vi "test-quintic-spline-05.vi"() -> (3 "Test Passed":bool)   [LabVIEW 2019]
uses:
  <vilib>/Rock Robotics/WPI/ThirdParty/JAS_Junk/TrajLib/POSEwCURVATURE.ctl
  <vilib>/Rock Robotics/WPI/ThirdParty/JAS_Junk/TrajLib/POSE2D.ctl
  <vilib>/Rock Robotics/WPI/ThirdParty/JAS_Junk/TrajLib/TRANSLATION2D.ctl
  <vilib>/Rock Robotics/WPI/ThirdParty/JAS_Junk/TrajLib/ROTATION2D.ctl
  <vilib>/Rock Robotics/WPI/ThirdParty/JAS_Junk/TrajLib/Rotation_CreateAngle.vi
  <vilib>/Rock Robotics/WPI/ThirdParty/JAS_Junk/TrajLib/Translation_Create.vi
  <vilib>/Rock Robotics/WPI/ThirdParty/JAS_Junk/TrajLib/Util_CalcDist.vi
  <vilib>/Rock Robotics/WPI/ThirdParty/JAS_Junk/TrajLib/Trajectory_Library.lvlib
panel:
  out "XY Graph":cluster{dbl[], dbl[]}(graph)
  out "Numb\nWaypoints":i32
  out "All Interior \nwayPoints\nFound (True)":bool
  out "end rot = 0":dbl
  out "end y = 0":dbl
  out "end x = 0":dbl
  out "start rot = 0":dbl
  out "start y = 0":dbl
  out "start x = 0":dbl
  out "max dtheta < 0.0872":dbl
  out "max dy < 0.00127":dbl
  out "max dx  < 0.127":dbl
  out "Overall Error":errorcluster
  out "Elements":i32
  out "Create Spline Error":errorcluster
  out "SplinePoses\nWCurve":T1[](array[typedef]) {"POSE"."ROTATION"."SIN" format="%13.4f"; "POSE"."ROTATION"."COS" format="%13.4f"; "POSE"."ROTATION"."VALUE" format="%13.4f"; "POSE"."TRANSLATION"."Y" format="%14.3f"; "POSE"."TRANSLATION"."X" format="%14.3f"}
  out "Elapsed Time":dbl
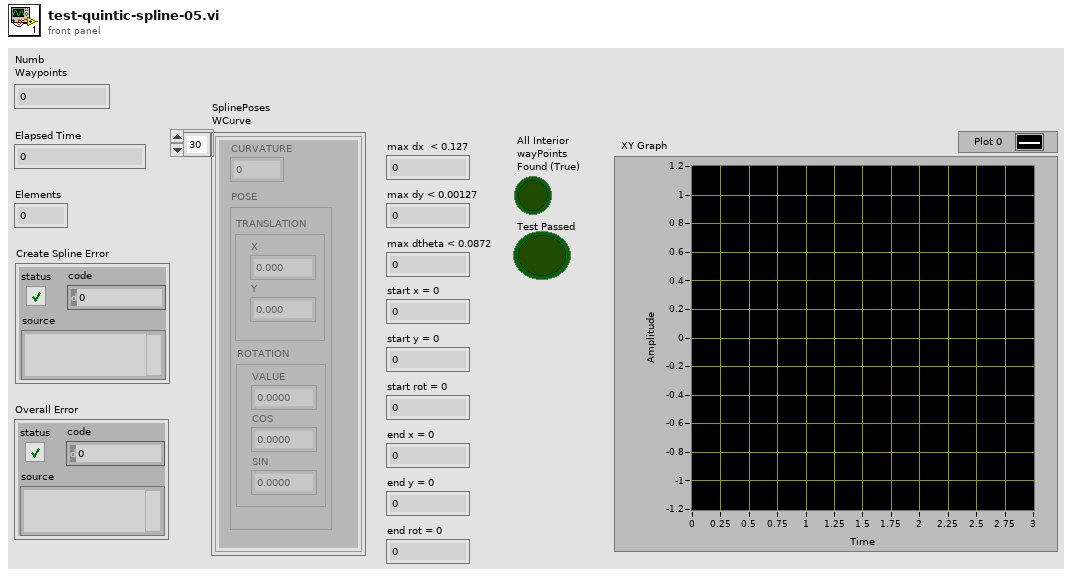
[diagram p1: front panel]
types:
  T1 = typedef "Trajectory_Library.lvlib/POSEwCURVATURE.ctl" = cluster{"CURVATURE":dbl, "POSE":T2}
  T2 = typedef "Trajectory_Library.lvlib/POSE2D.ctl" = cluster{"TRANSLATION":T3, "ROTATION":T4}
  T3 = typedef "Trajectory_Library.lvlib/TRANSLATION2D.ctl" = cluster{"X":dbl, "Y":dbl}
  T4 = typedef "Trajectory_Library.lvlib/ROTATION2D.ctl" = cluster{"VALUE":dbl, "COS":dbl, "SIN":dbl}
  T5 = typedef "Trajectory_Library.lvlib/SPLINE_CTRL_VECTOR.ctl" = cluster{"Xs":dbl[], "Ys":dbl[]}
  T6 = typedef "Trajectory_Library.lvlib/SPLINE.ctl" = cluster{"Degree":i32, "Coefficients":T7}
  T7 = typedef "NI_Matrix.lvlib/RealMatrix.ctl" = dbl[][]
  T8 = typedef "Trajectory_Library.lvlib/TWIST2D.ctl" = cluster{"dX":dbl, "dY":dbl, "dTHETA":dbl}
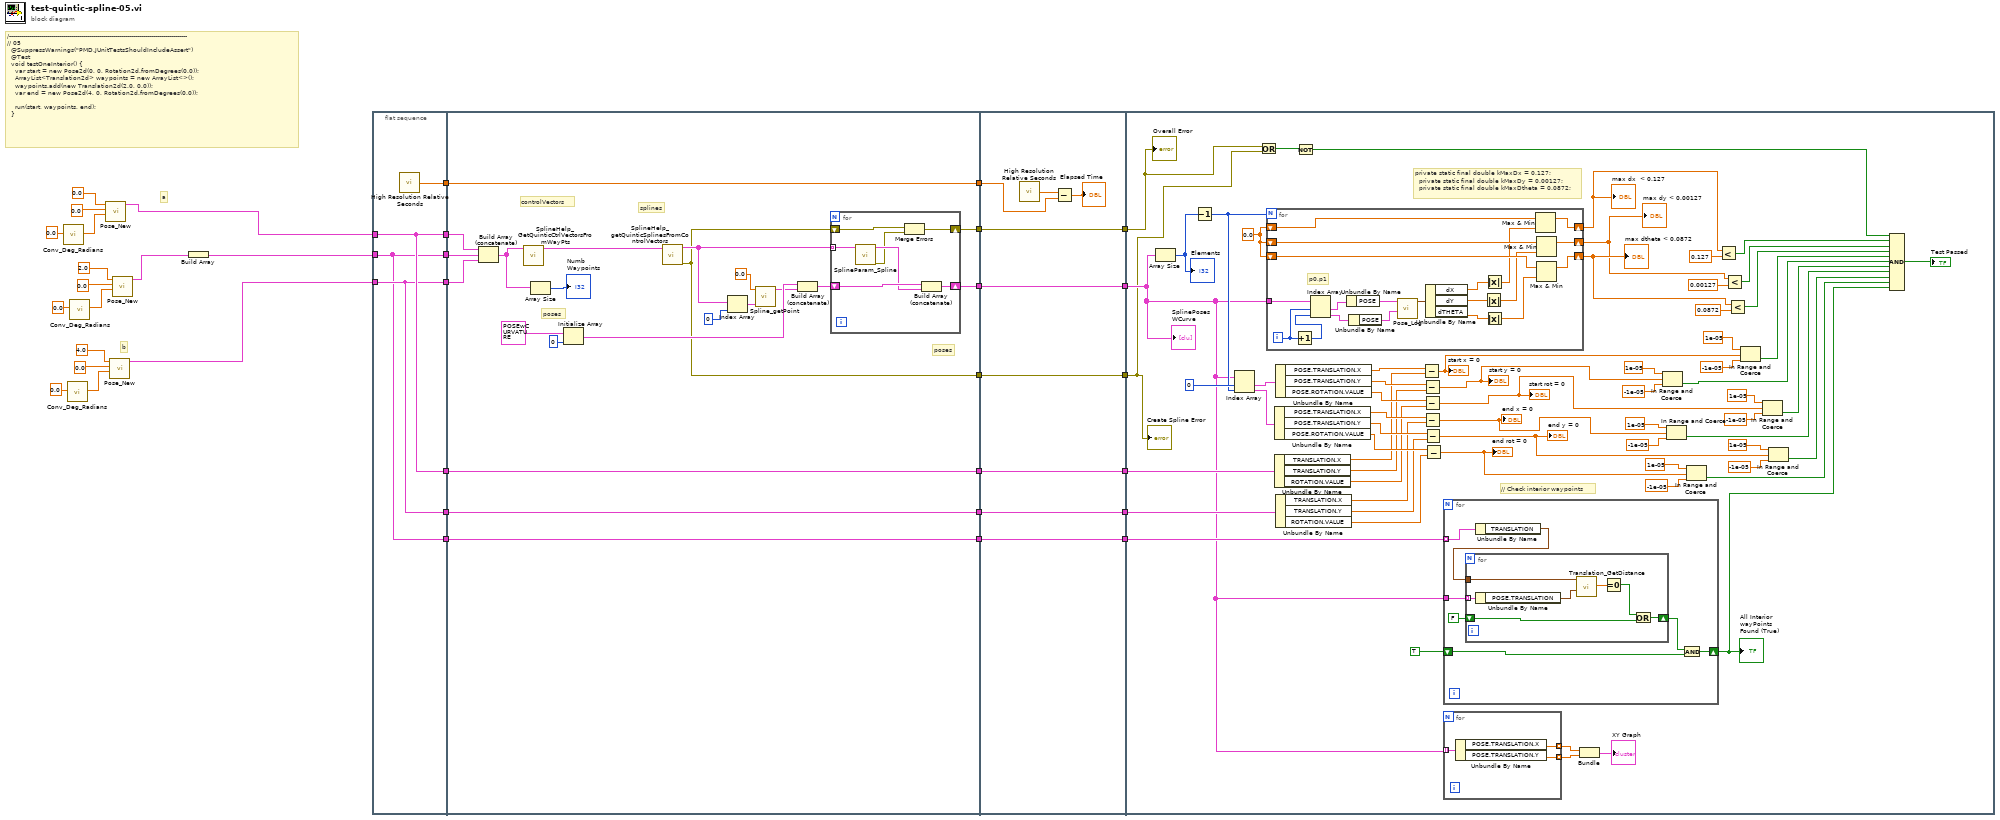
[diagram p0: block diagram]
diagram:
  # "b"
  # "a"
  # "/-----------------------------------------------------------------------------------------\n// 05\n  @SuppressWarnings(\"PMD.JUnitTestsShouldIncludeAssert\")\n  @Test\n  void testOneInterior() {\n    var start = new Pose2d(0, 0, Rotation2d.fromDegrees(0.0));\n    ArrayList<Translation2d> waypoints = new ArrayList<>();\n    waypoints.add(new Translation2d(2.0, 0.0));\n    var end = new Pose2d(4, 0, Rotation2d.fromDegrees(0.0));\n\n    run(start, waypoints, end);\n  }"
  n1 = call <vilib>:"Conv_Deg_Radians.vi"("Degress"=0.0) -> ("Radians"=w11:dbl)  [unwired: 10 in]
  n2 = call <vilib>:"Conv_Deg_Radians.vi"("Degress"=0.0) -> ("Radians"=w14:dbl)  [unwired: 10 in]
  n3 = call <vilib>:"Conv_Deg_Radians.vi"("Degress"=0.0) -> ("Radians"=w6:dbl)  [unwired: 10 in]
  n4 = call <vilib>:"Pose_New.vi"("Heading"=w11, "Y"=0.0, "X"=0.0) -> ("out POSe"=w2:T2)  [unwired: 8 in]
  n5 = call <vilib>:"Pose_New.vi"("Heading"=w14, "Y"=0.0, "X"=4.0) -> ("out POSe"=w1:T2)  [unwired: 8 in]
  n6 = call <vilib>:"Pose_New.vi"("Heading"=w6, "Y"=0.0, "X"=2.0) -> ("out POSe"=w4:T2)  [unwired: 8 in]
  n7 = Build Array(w4) -> (w3:T2[])
  n8 = flat-sequence {
    tunnel: w2 -> [w39]
    tunnel: [w39] -> w36
    tunnel: w1 -> [w38]
    tunnel: [w38] -> w35
    tunnel: [w40] -> w34
    tunnel: [w39] -> w26
    tunnel: [w38] -> w23
    tunnel: [w37] -> w18
    tunnel: w3 -> [w37]
    tunnel: [w37] -> w17
    tunnel: w36 -> [w46]
    tunnel: w35 -> [w44]
    tunnel: [w62] -> w33
    tunnel: w34 -> [w62]
    tunnel: [w52] -> w32
    tunnel: [w51] -> w30
    tunnel: [w50] -> w28
    tunnel: w26 -> [w49]
    tunnel: [w49] -> w25
    tunnel: w23 -> [w48]
    tunnel: [w48] -> w22
    tunnel: [w47] -> w19
    tunnel: w18 -> [w47]
    tunnel: w17 -> [w41]
    tunnel: w33 -> [w78]
    tunnel: w32 -> [w77]
    tunnel: [w77] -> w31
    tunnel: w30 -> [w76]
    tunnel: [w76] -> w29
    tunnel: w28 -> [w75]
    tunnel: [w75] -> w27
    tunnel: w25 -> [w72]
    tunnel: [w72] -> w24
    tunnel: w22 -> [w71]
    tunnel: [w71] -> w21
    tunnel: [w70] -> w20
    tunnel: w19 -> [w70]
    tunnel: w31 -> [w119]
    tunnel: w29 -> [w107]
    tunnel: w27 -> [w106]
    tunnel: w24 -> [w141]
    tunnel: w21 -> [w140]
    tunnel: w20 -> [w123]
    frame #0 {
      n9 = call <vilib>:"High Resolution Relative Seconds.vi"() -> ("relative seconds"=w40:dbl)
    }
    frame #1 {
      # "poses"
      # "poses"
      # "splines"
      # "controlVectors"
      n10 = Build Array (concatenate)(w46, w41, w44) -> (w43:T2[])
      n11 = call <vilib>:"SplineHelp_GetQuinticCtrlVectorsFromWayPts.vi"("WayPoints"=w43) -> ("SplineControlVectors"=w45:T5[])  [unwired: 10 in]
      n12 = Array Size(array=w43) -> (size(s)=→"Numb\nWaypoints":i32)
      n13 = Initialize Array(T1 {"CURVATURE"=0.0, "POSE"={"TRANSLATION"={"X"=0.0, "Y"=0.0}, "ROTATION"={"VALUE"=0.0, "COS"=1.0, "SIN"=0.0}}} ("POSEwCURVATURE"), 0 ("dimension size")) -> (w56:T1[])
      n14 = call <vilib>:"SplineHelp_getQuinticSplinesFromControlVectors.vi"("ControlVectors"=w45) -> ("error out"=w51:errorcluster, "splines"=w53:T6[])  [unwired: 9 in]
      n15 = Index Array(array=w53, index=0) -> (element=w58:T6)
      n16 = call <vilib>:"Spline_getPoint.vi"("inputSPLINE"=w58, "Time"=0.0) -> ("POSEwCURVATURE"=w55:T1)  [unwired: 9 in]
      n17 = Build Array (concatenate)(w56, w55) -> (w54:T1[])
      n18 = for {
        shift-right: [w66] -> w52
        shift-left: w54 -> [w68]
        tunnel: w53 -> [w69] mode=indexing
        shift-right: [w64] -> w50
        shift-left: w51 -> [w65]
        n19 = call <vilib>:"SplineParam_Spline.vi"("inputSPLINE"=w69) -> ("error out"=w63:errorcluster, "outputPOSEwCURVATURE"=w67:T1[])  [unwired: 9 in]
        n20 = Merge Errors(w65, w63) -> (w64:errorcluster)
        n21 = Build Array (concatenate)(w68, w67) -> (w66:T1[])
      }
    }
    frame #2 {
      n22 = call <vilib>:"High Resolution Relative Seconds.vi"() -> ("relative seconds"=w73:dbl)
      n23 = Subtract(x=w73, y=w78) -> (x-y=→"Elapsed Time":dbl)
    }
    frame #3 {
      w142 = 0.0
      # "// Check interior waypoints"
      # "private static final double kMaxDx = 0.127;\n  private static final double kMaxDy = 0.00127;\n  private static final double kMaxDtheta = 0.0872;"
      n24 = Array Size(array=w119) -> (size(s)=w143:i32)
      "Elements" <- w143
      n25 = Decrement(x=w143) -> (x-1=w138:i32)
      n26 = Index Array(array=w119, index #1=0 ("index"), index #2=w138) -> (element #1=w137:T1, element #2=w136:T1)
      n27 = Or(x=w106, y=w107) -> (x .or. y?=w108:bool)
      n28 = for {
        N: w138 -> [_]
        tunnel: w119 -> [w178]
        shift-right: [w169] -> w112
        shift-left: w142 -> [w166]
        shift-right: [w167] -> w114
        shift-left: w142 -> [w164]
        shift-right: [w168] -> w113
        shift-left: w142 -> [w165]
        i -> [w180]
        # "p0,p1"
        n29 = Increment(x=w180) -> (x+1=w179:i32)
        n30 = Index Array(array=w178, index #1=w180, index #2=w179) -> (element #1=w177:T1, element #2=w176:T1)
        n31 = Unbundle By Name(w177) -> ("POSE"=w175:T2)
        n32 = Unbundle By Name(w176) -> ("POSE"=w174:T2)
        n33 = call <vilib>:"Pose_Log.vi"("end POSE"=w174, "in POSE"=w175) -> ("out TWIST"=w173:T8)  [unwired: 9 in]
        n34 = Unbundle By Name(w173) -> ("dX"=w170:dbl, "dY"=w171:dbl, "dTHETA"=w172:dbl)
        n35 = Absolute Value(x=w171) -> (abs(x)=w162:dbl)
        n36 = Absolute Value(x=w170) -> (abs(x)=w163:dbl)
        n37 = Absolute Value(x=w172) -> (abs(x)=w161:dbl)
        n38 = Max & Min(x=w166, y=w163) -> (max(x,y)=w169:dbl)  [unwired: 1 out]
        n39 = Max & Min(x=w165, y=w162) -> (max(x,y)=w168:dbl)  [unwired: 1 out]
        n40 = Max & Min(x=w164, y=w161) -> (max(x,y)=w167:dbl)  [unwired: 1 out]
      }
      "max dx  < 0.127" <- w112
      "max dy < 0.00127" <- w113
      "max dtheta < 0.0872" <- w114
      n41 = Unbundle By Name(w136) -> ("POSE.TRANSLATION.X"=w132:dbl, "POSE.TRANSLATION.Y"=w131:dbl, "POSE.ROTATION.VALUE"=w130:dbl)
      n42 = Unbundle By Name(w141) -> ("TRANSLATION.X"=w129:dbl, "TRANSLATION.Y"=w128:dbl, "ROTATION.VALUE"=w127:dbl)
      n43 = Unbundle By Name(w137) -> ("POSE.TRANSLATION.X"=w135:dbl, "POSE.TRANSLATION.Y"=w134:dbl, "POSE.ROTATION.VALUE"=w133:dbl)
      n44 = Unbundle By Name(w140) -> ("TRANSLATION.X"=w126:dbl, "TRANSLATION.Y"=w125:dbl, "ROTATION.VALUE"=w124:dbl)
      n45 = Not(x=w108) -> (.not. x?=w105:bool)
      n46 = Subtract(x=w135, y=w129) -> (x-y=w101:dbl)
      "start x = 0" <- w101
      n47 = Subtract(x=w134, y=w128) -> (x-y=w80:dbl)
      "start y = 0" <- w80
      n48 = Subtract(x=w133, y=w127) -> (x-y=w84:dbl)
      "start rot = 0" <- w84
      n49 = Subtract(x=w132, y=w126) -> (x-y=w85:dbl)
      "end x = 0" <- w85
      n50 = Subtract(x=w131, y=w125) -> (x-y=w92:dbl)
      "end y = 0" <- w92
      n51 = Subtract(x=w130, y=w124) -> (x-y=w96:dbl)
      "end rot = 0" <- w96
      n52 = for {
        tunnel: w123 -> [w148] mode=indexing
        tunnel: w119 -> [w153]
        shift-right: [w152] -> w104
        shift-left: TRUE -> [w151]
        n53 = Unbundle By Name(w148) -> ("TRANSLATION"=w147:T3)
        n54 = for {
          tunnel: w153 -> [w157] mode=indexing
          shift-right: [w160] -> w149
          shift-left: FALSE -> [w159]
          tunnel: w147 -> [w158]
          n55 = Unbundle By Name(w157) -> ("POSE.TRANSLATION"=w156:T3)
          n56 = call <vilib>:"Translation_GetDistance.vi"("other Translation"=w156, "In Translation"=w158) -> ("Distance"=w155:dbl)  [unwired: 9 in]
          n57 = Equal To 0?(x=w155) -> (x = 0?=w154:bool)
          n58 = Or(x=w154, y=w159) -> (x .or. y?=w160:bool)
        }
        n59 = And(x=w149, y=w151) -> (x .and. y?=w152:bool)
      }
      "All Interior \nwayPoints\nFound (True)" <- w104
      n60 = for {
        tunnel: [w146] -> w121 mode=indexing
        tunnel: [w145] -> w120 mode=indexing
        tunnel: w119 -> [w144] mode=indexing
        n61 = Unbundle By Name(w144) -> ("POSE.TRANSLATION.X"=w146:dbl, "POSE.TRANSLATION.Y"=w145:dbl)
      }
      n62 = Bundle(w121, w120) -> (→"XY Graph":cluster{dbl[], dbl[]})  [unwired: 1 in]
      n63 = In Range and Coerce(upper limit=1e-05, x=w80, lower limit=-1e-05) -> (In Range?=w81:bool)  [unwired: 1 out]
      n64 = In Range and Coerce(upper limit=1e-05, x=w85, lower limit=-1e-05) -> (In Range?=w87:bool)  [unwired: 1 out]
      n65 = In Range and Coerce(upper limit=1e-05, x=w96, lower limit=-1e-05) -> (In Range?=w97:bool)  [unwired: 1 out]
      n66 = Less?(x=w112, y=0.127) -> (x < y?=w111:bool)
      n67 = Less?(x=w113, y=0.00127) -> (x < y?=w110:bool)
      n68 = Less?(x=w114, y=0.0872) -> (x < y?=w109:bool)
      n69 = In Range and Coerce(upper limit=1e-05, x=w101, lower limit=-1e-05) -> (In Range?=w100:bool)  [unwired: 1 out]
      n70 = In Range and Coerce(upper limit=1e-05, x=w84, lower limit=-1e-05) -> (In Range?=w86:bool)  [unwired: 1 out]
      n71 = In Range and Coerce(upper limit=1e-05, x=w92, lower limit=-1e-05) -> (In Range?=w93:bool)  [unwired: 1 out]
      n72 = Compound Arithmetic op=AND(w105, w111, w110, w109, w100, w81, w86, w87, w93, w97, w104) -> (→"Test Passed":bool)
      "SplinePoses\nWCurve" <- w119
      "Create Spline Error" <- w107
      "Overall Error" <- w106
    }
  }
